vi "WPI_AccelerometerInternalOpen.vi"(8 "error in":errorcluster, 9 "Accel Range":T9) -> (0 "error out":errorcluster, 3 "AccelerometerDevRef":T1={"DevStatus"={"status"=FALSE, "code"=0, "source"=""}, "Scaling"={"Gain (VoltsPerG)"=0.0, "Center Voltage"=0.0}, "Analog Channels"={"X-Axis"=enum."Invalid", "Y-Axis"=enum."Invalid", "Z-Axis"=enum."Invalid"}, "I2C Bus"=enum."Invalid", "SPI Bus"=enum."Invalid", "Accel Range"=0, "ADXL Axes"={"X-Axis"=FALSE, "Y-Axis"=FALSE, "Z-Axis"=FALSE}, "Handle"=0, "Device Address"=0, "Accel Type"=enum."Analog"} {"Device Address" format="%.0x"; "Accel Range" items=["+/- 2 g", "+/- 4 g", "+/- 8 g", "+/- 16 g"]})   [LabVIEW 2017]
doc: "Opens a reference to the accelerometer you specify. You must open a reference before using any other VIs on this palette.\n\nThis software is licensed. Open the labview\\readme\\WPI Robotics Library Open Source License.txt file for more information."
uses:
  <vilib>/Rock Robotics/WPI/Accelerometer/WPI_AccelerometerRange.ctl
  <vilib>/Rock Robotics/WPI/Accelerometer/WPI_AccelerometerDevRef.ctl
  <vilib>/Rock Robotics/WPI/Accelerometer/WPI_AccelerometerScaling.ctl
  <vilib>/Rock Robotics/WPI/Accelerometer/WPI_AccelerometerAnalogChannels.ctl
  <vilib>/Rock Robotics/SystemInterfaces/AI/FPGA_AIChannel.ctl
  <vilib>/Rock Robotics/SystemInterfaces/i2clib/i2c_bus.ctl
  <vilib>/Rock Robotics/SystemInterfaces/spilib/spi_bus.ctl
  <vilib>/Rock Robotics/WPI/Accelerometer/ADXL345 Range.ctl
  <vilib>/Rock Robotics/WPI/Accelerometer/WPI_AccelerometerADXL345 Axes.ctl
  <vilib>/Rock Robotics/WPI/Accelerometer/InternalAccelerometer/WPI_Accelerometer_Internal_MMA8452Q_Registers.ctl
panel:
  # "ADXL"
  # "Analog"
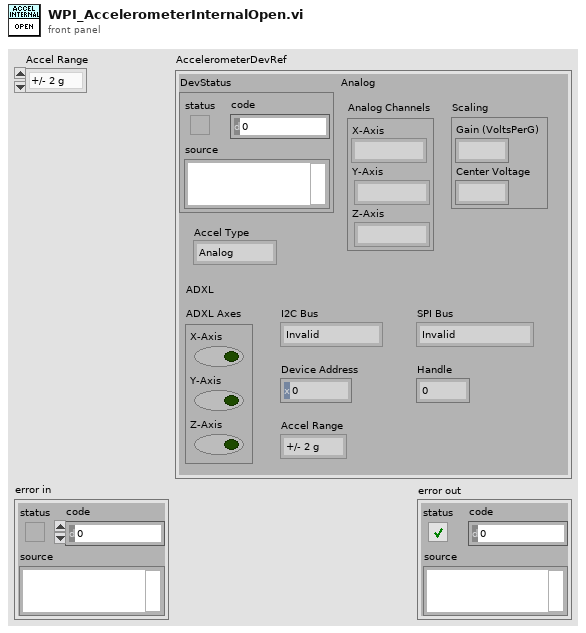
[diagram p1: front panel]
types:
  T1 = typedef "WPI_AccelerometerDevRef.ctl" = cluster{"DevStatus":errorcluster, "Scaling":T2, "Analog Channels":T3, "I2C Bus":T5, "SPI Bus":T6, "Accel Range":T7, "ADXL Axes":T8, "Handle":i32, "Device Address":u8, "Accel Type":enum16{"Analog", "ADXL345 I2C", "ADXL345 SPI", "Internal", "ADXL362 SPI"}}
  T2 = typedef "WPI_AccelerometerScaling.ctl" = cluster{"Gain (VoltsPerG)":dbl, "Center Voltage":dbl}
  T3 = typedef "WPI_AccelerometerAnalogChannels.ctl" = cluster{"X-Axis":T4, "Y-Axis":T4, "Z-Axis":T4}
  T4 = typedef "FPGA_AIChannel.ctl" = enum8{"AI 0", "AI 1", "AI 2", "AI 3", "AI MXP 0", "AI MXP 1", "AI MXP 2", "AI MXP 3", "Invalid"}
  T5 = typedef "i2c_bus.ctl" = enum16{"I2C On-Board", "I2C MXP", "Invalid"}
  T6 = typedef "spi_bus.ctl" = enum16{"SPI On-Board, CS0", "SPI On-Board, CS1", "SPI On-Board, CS2", "SPI On-Board, CS3", "SPI MXP", "Invalid"}
  T7 = typedef "ADXL345 Range.ctl" = u8
  T8 = typedef "WPI_AccelerometerADXL345 Axes.ctl" = cluster{"X-Axis":bool, "Y-Axis":bool, "Z-Axis":bool}
  T9 = typedef "WPI_AccelerometerRange.ctl" = enum16{"+/- 2 g", "+/- 4 g", "+/- 8 g"}
  T10 = typedef "WPI_Accelerometer_Internal_MMA8452Q_Registers.ctl" = u8
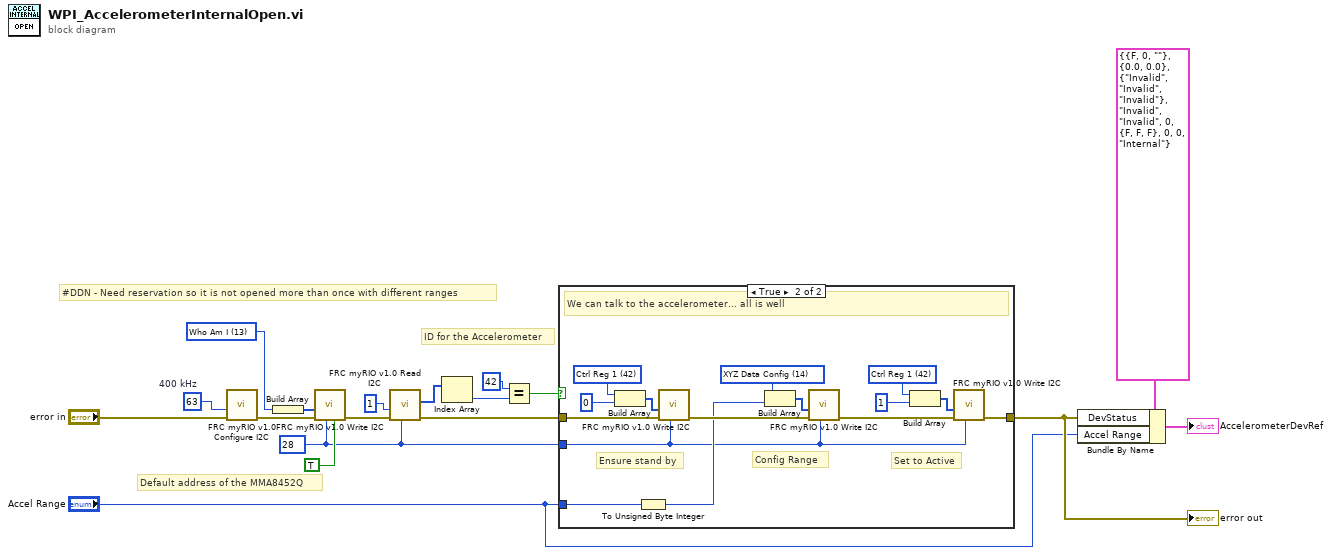
[diagram p0: block diagram]
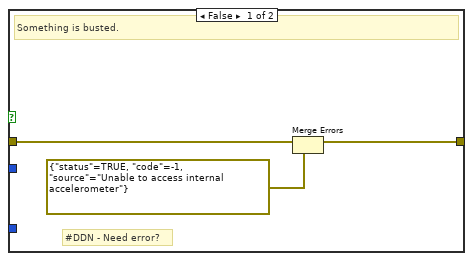
[diagram p2: hidden frame]
diagram:
  w16 = T10 13 items=["Status"=0, "Out X MSB"=1, "Out X LSB"=2, "Out Y MSB"=3, "Out Y LSB"=4, "Out Z MSB"=5, "Out Z LSB"=6, "Who Am I"=13, "XYZ Data Config"=14, "Ctrl Reg 1"=42]
  w5 = u8 28 ("Accel.ADDR")
  w18 = u8 63  # 400 kHz
  # "#DDN - Need reservation so it is not opened more than once with different ranges"
  # "ID for the Accelerometer"
  # "Default address of the MMA8452Q"
  n1 = call <vilib>:"FRC myRIO v1.0 Configure I2C.vi"("error in (no error)"="error in", "I2C Counter Value"=w18) -> ("error out"=w17:errorcluster)  [unwired: 9 in]
  n2 = Build Array(w16) -> (w15:T10[])
  n3 = call <vilib>:"FRC myRIO v1.0 Write I2C.vi"("Keep Bus Busy"=TRUE, "Slave Address (7-bit)"=w5, "Error In (No Error)"=w17, "Data to Write"=w15) -> ("error out"=w13:errorcluster)  [unwired: 7 in]
  n4 = call <vilib>:"FRC myRIO v1.0 Read I2C.vi"("Slave Address (7-bit)"=w5, "Error In (No Error)"=w13, "Bytes to Read"=u32 1) -> ("error out"=w7:errorcluster, "Data Read"=w11:u8[])  [unwired: 7 in]
  n5 = Index Array(array=w11) -> (element=w10:u8)  [unwired: 1 in]
  n6 = Equal?(x=u8 42 ("y"), y=w10) -> (x = y?=w8:bool)
  n7 = case shown="True" w8 {
    tunnel: w7 -> [w19 w35]
    tunnel: [w20 w22] -> w3
    tunnel: "Accel Range" -> [_ w29]
    tunnel: w5 -> [_ w23]
    frame False {
      # "#DDN - Need error?"
      # "Something is busted."
      n8 = Merge Errors(w19, errorcluster {"status"=TRUE, "code"=-1, "source"="Unable to access internal accelerometer"} ("error out")) -> (w20:errorcluster)
    }
    frame True {
      w26 = T10 42 items=["Status"=0, "Out X MSB"=1, "Out X LSB"=2, "Out Y MSB"=3, "Out Y LSB"=4, "Out Z MSB"=5, "Out Z LSB"=6, "Who Am I"=13, "XYZ Data Config"=14, "Ctrl Reg 1"=42]
      w32 = T10 14 items=["Status"=0, "Out X MSB"=1, "Out X LSB"=2, "Out Y MSB"=3, "Out Y LSB"=4, "Out Z MSB"=5, "Out Z LSB"=6, "Who Am I"=13, "XYZ Data Config"=14, "Ctrl Reg 1"=42]
      w34 = T10 42 items=["Status"=0, "Out X MSB"=1, "Out X LSB"=2, "Out Y MSB"=3, "Out Y LSB"=4, "Out Z MSB"=5, "Out Z LSB"=6, "Who Am I"=13, "XYZ Data Config"=14, "Ctrl Reg 1"=42]
      # "Set to Active"
      # "Config Range"
      # "Ensure stand by"
      # "We can talk to the accelerometer... all is well"
      n9 = Build Array(w34, u8 0) -> (w36:T10[])
      n10 = To Unsigned Byte Integer(number=w29) -> (unsigned 8bit integer=w28:u8)
      n11 = call <vilib>:"FRC myRIO v1.0 Write I2C.vi"("Slave Address (7-bit)"=w23, "Error In (No Error)"=w35, "Data to Write"=w36) -> ("error out"=w30:errorcluster)  [unwired: 8 in]
      n12 = Build Array(w32, w28) -> (w31:T10[])
      n13 = call <vilib>:"FRC myRIO v1.0 Write I2C.vi"("Slave Address (7-bit)"=w23, "Error In (No Error)"=w30, "Data to Write"=w31) -> ("error out"=w24:errorcluster)  [unwired: 8 in]
      n14 = Build Array(w26, u8 1) -> (w25:T10[])
      n15 = call <vilib>:"FRC myRIO v1.0 Write I2C.vi"("Slave Address (7-bit)"=w23, "Error In (No Error)"=w24, "Data to Write"=w25) -> ("error out"=w22:errorcluster)  [unwired: 8 in]
    }
  }
  "error out" <- w3
  n16 = Bundle By Name(cluster=T1 {"DevStatus"={"status"=FALSE, "code"=0, "source"=""}, "Scaling"={"Gain (VoltsPerG)"=0.0, "Center Voltage"=0.0}, "Analog Channels"={"X-Axis"=enum."Invalid", "Y-Axis"=enum."Invalid", "Z-Axis"=enum."Invalid"}, "I2C Bus"=enum."Invalid", "SPI Bus"=enum."Invalid", "Accel Range"=0, "ADXL Axes"={"X-Axis"=FALSE, "Y-Axis"=FALSE, "Z-Axis"=FALSE}, "Handle"=0, "Device Address"=0, "Accel Type"=enum."Internal"} ("AccelerometerDevRef"), "DevStatus"=w3, "Accel Range"="Accel Range") -> (→"AccelerometerDevRef":T1)
